vi "Read Inventory.vi"(8 "error in (no error)":errorcluster, 11 "Productos in":refnum<class "Productos.lvclass">) -> (0 "error out":errorcluster, 3 "Productos out":refnum<class "Productos.lvclass">)   [LabVIEW 2020, in "Productos.lvlib" / "Productos.lvclass"]
uses:
  Productos.lvclass
  Productos.lvclass/Productos.ctl
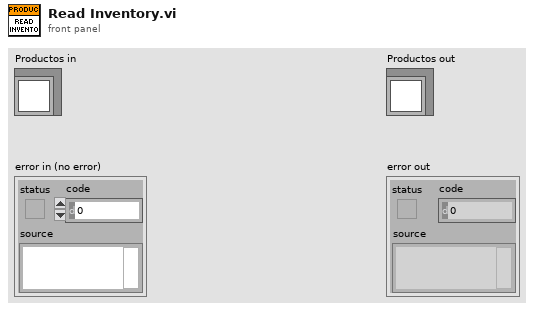
[diagram p1: front panel]
types:
  T1 = enum16{"open", "replace", "create", "open or create", "replace or create", "replace or create with confirmation"}
  T2 = cluster{"[0]":string, "[1]":string, "[2]":string, "[3]":string, "[4]":string, "[5]":string, "[6]":string, "[7]":string, "[8]":string}
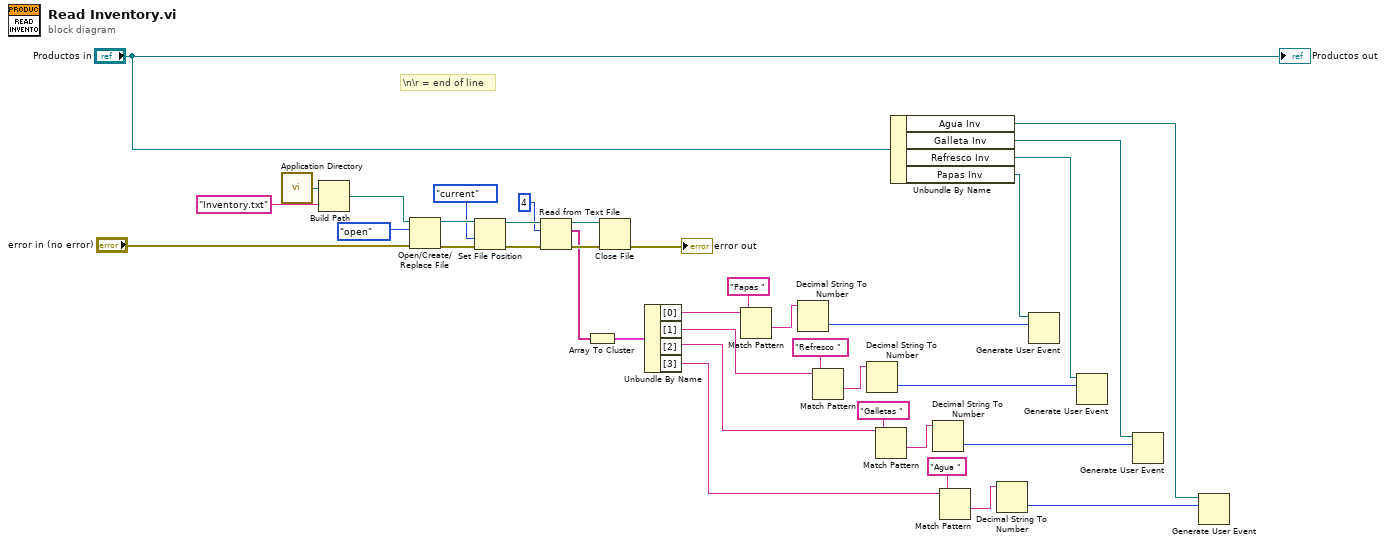
[diagram p0: block diagram]
diagram:
  # "\\n\\r = end of line"
  n1 = call <vilib>:"Application Directory.vi"() -> ("Application Directory"=w30:path)
  n2 = Build Path(base path=w30, name or relative path="Inventory.txt") -> (appended path=w37:path)
  n3 = Open/Create/Replace File(file path (use dialog)=w37, error in="error in (no error)", operation (0:open)=T1."open") -> (refnum out=w33:refnum<file>, error out=w35:errorcluster)  [unwired: 3 in, 1 out]
  n4 = Set File Position(refnum=w33, from (0:start)=enum16{"start", "end", "current"}."current", error in=w35) -> (refnum out=w32:refnum<file>, error out=w28:errorcluster)  [unwired: 1 in]
  n5 = Read from Text File(file (use dialog)=w32, count=4, error in=w28) -> (refnum out=w27:refnum<file>, text=w10:string[], error out=w29:errorcluster)  [unwired: 1 in, 1 out]
  n6 = Array To Cluster(array=w10) -> (cluster=w11:T2)
  n7 = Close File(refnum=w27, error in=w29) -> (error out=→"error out":errorcluster)  [unwired: 1 out]
  n8 = Unbundle By Name(w11) -> ("[0]"=w12:string, "[1]"=w21:string, "[2]"=w22:string, "[3]"=w23:string)
  n9 = Match Pattern(string=w12, regular expression="Papas ") -> (after substring=w14:string)  [unwired: 1 in, 3 out]
  n10 = Decimal String To Number(string=w14) -> (number=w4:i32)  [unwired: 2 in, 1 out]
  n11 = Match Pattern(string=w21, regular expression="Refresco ") -> (after substring=w15:string)  [unwired: 1 in, 3 out]
  n12 = Decimal String To Number(string=w15) -> (number=w3:i32)  [unwired: 2 in, 1 out]
  n13 = Match Pattern(string=w22, regular expression="Galletas ") -> (after substring=w18:string)  [unwired: 1 in, 3 out]
  n14 = Unbundle By Name("Productos in") -> ("Agua Inv"=w8:refnum<user-event>, "Galleta Inv"=w7:refnum<user-event>, "Refresco Inv"=w6:refnum<user-event>, "Papas Inv"=w5:refnum<user-event>)
  n15 = Decimal String To Number(string=w18) -> (number=w2:i32)  [unwired: 2 in, 1 out]
  n16 = Match Pattern(string=w23, regular expression="Agua ") -> (after substring=w19:string)  [unwired: 1 in, 3 out]
  n17 = Decimal String To Number(string=w19) -> (number=w1:i32)  [unwired: 2 in, 1 out]
  n18 = Generate User Event(user event=w5, event data cluster=w4) -> ()  [unwired: 2 in, 2 out]
  n19 = Generate User Event(user event=w6, event data cluster=w3) -> ()  [unwired: 2 in, 2 out]
  n20 = Generate User Event(user event=w7, event data cluster=w2) -> ()  [unwired: 2 in, 2 out]
  n21 = Generate User Event(user event=w8, event data cluster=w1) -> ()  [unwired: 2 in, 2 out]
  "Productos out" <- "Productos in"
